vi "Add File to Tree.vi"(4 "Hide Undefined Channels":bool, 5 "Relative File Path":string, 6 "Filter Settings":T1={"Filtered Groups"=[], "Group Filter Mode"=enum."Exclude", "Group Filter Regex?"=FALSE, "Filtered Channels"=[], "Channel Filter Mode"=enum."Exclude", "Channel Filter Regex?"=FALSE, "Filter Time Start"=timestamp(0 s since 1904-01-01), "Filter Time End"=timestamp(0 s since 1904-01-01), "Time Filter Mode"=enum."Include", "Time Filter Enabled"=FALSE}, 7 "Hierarchy":string[](array[string]), 8 "error in (no error)":errorcluster, 9 "Tree Items Created In":variant, 10 "File Path":path, 11 "TreeControl in":refnum<vi>) -> (0 "error out":errorcluster, 1 "Tree Items Created Out":variant)   [LabVIEW 2017, in "XTree.xctl"]
doc: "Adds a single file to the tree. A variant is used to keep track of tree locations which have been created."
uses:
  <vilib>/addons/_NIFileIO/XTree/XTree.xctl
  <vilib>/addons/_NIFileIO/XTree/Controls/Filter Settings.ctl
  <vilib>/addons/_NIFileIO/XTree/Controls/Filter Mode.ctl
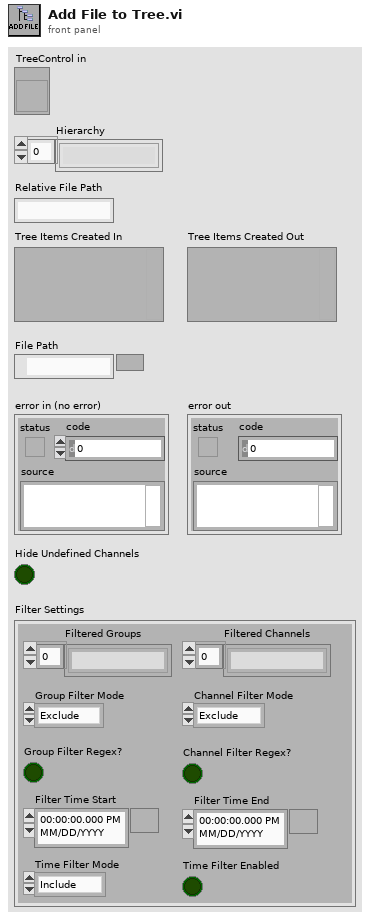
[diagram p1: front panel]
types:
  T1 = typedef "XTree.xctl/Filter Settings.ctl" = cluster{"Filtered Groups":string[], "Group Filter Mode":T2, "Group Filter Regex?":bool, "Filtered Channels":string[], "Channel Filter Mode":T2, "Channel Filter Regex?":bool, "Filter Time Start":timestamp, "Filter Time End":timestamp, "Time Filter Mode":T2, "Time Filter Enabled":bool}
  T2 = typedef "XTree.xctl/Filter Mode.ctl" = enum16{"Exclude", "Include"}
  T3 = enum16{"open", "open or create", "create or replace", "create", "open (read-only)"}
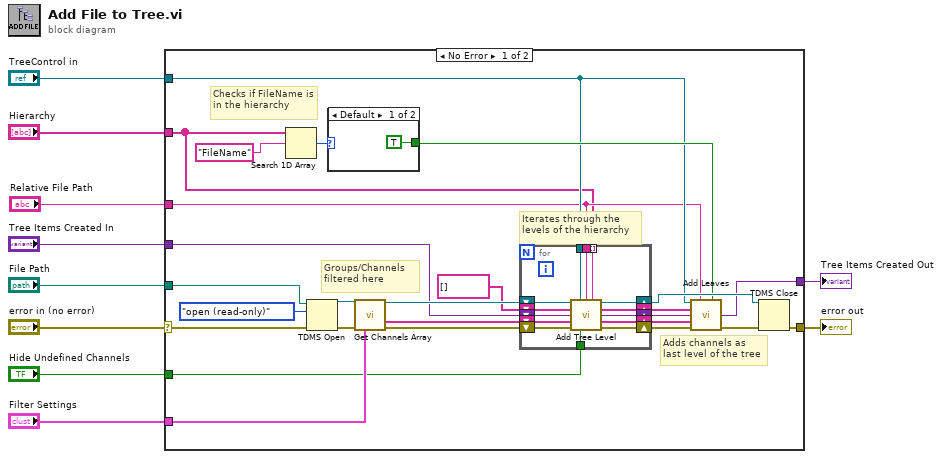
[diagram p0: block diagram]
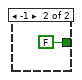
[diagram p2: hidden frame]
diagram:
  n1 = case shown="No Error" "error in (no error)" {
    selector: "error in (no error)" -> [w28 w54]
    tunnel: [w27 w54] -> w9
    tunnel: [w17 w53] -> w2
    tunnel: "Tree Items Created In" -> [w26 w53]
    tunnel: "File Path" -> [w14 _]
    tunnel: "Hierarchy" -> [w11 _]
    tunnel: "TreeControl in" -> [w19 _]
    tunnel: "Filter Settings" -> [w16 _]
    tunnel: "Hide Undefined Channels" -> [w15 _]
    tunnel: "Relative File Path" -> [w12 _]
    frame No Error {
      # "Groups/Channels filtered here"
      # "Adds channels as last level of the tree"
      # "Iterates through the levels of the hierarchy"
      # "Checks if FileName is in the hierarchy"
      n2 = Search 1D Array(1D array=w11, element="FileName") -> (index of element=w21:i32)  [unwired: 1 in]
      n3 = TDMS Open(8:w28, 10:T3."open (read-only)" ("operation (0:open)"), 11:w14) -> (0:w33:errorcluster, 3:w32:refnum<k34>)  [unwired: 4 in]
      n4 = case shown="Default" w21 {
        tunnel: [TRUE FALSE] -> w20
        frame Default {
        }
        frame -1 {
        }
      }
      n5 = call <vilib>:"Get Channels Array.vi"("TDMS File Reference in"=w32, "error in (no error)"=w33, "Filtering Settings"=w16) -> ("TDMS File Reference out"=w34:refnum<k34>, "Group/Channel Names"=w36:string[], "error out"=w13:errorcluster)  [unwired: 10 in]
      n6 = for {
        tunnel: w19 -> [w45]
        tunnel: w11 -> [w44] mode=indexing
        tunnel: w15 -> [w41]
        shift-right: [w52] -> w35
        shift-left: w34 -> [w49]
        shift-right: [w42] -> w24
        shift-left: string[] [] -> [w48]
        shift-right: [w46] -> w23
        shift-left: w26 -> [w47]
        shift-right: [w40] -> w18
        shift-left: w36 -> [w43]
        shift-right: [w50] -> w29
        shift-left: w13 -> [w51]
        tunnel: w12 -> [w39]
        n7 = call <vilib>:"Add Tree Level.vi"("tdms file"=w49, "Tree Refnum"=w45, "Relative File Path"=w39, "Property Name"=w44, "Tree Parent Tags In"=w48, "Tree Items Created In"=w47, "Group/Channel Names In"=w43, "error in (no error)"=w51, "Hide Undefined Channels"=w41) -> ("tdms file out"=w52:refnum<k34>, "Tree Parent Tags Out"=w42:string[], "Tree Items Created Out"=w46:variant, "Group/Channel Names Out"=w40:string[], "error out"=w50:errorcluster)  [unwired: 2 in]
      }
      n8 = call <vilib>:"Add Leaves.vi"("TreeControl in"=w19, "Relative File Path"=w12, "FileName In Hierarchy?"=w20, "Tree Parent Tags"=w24, "Tree Items Created In"=w23, "Group/Channel Names"=w18, "error in (no error)"=w29) -> ("Tree Items Created Out"=w17:variant, "error out"=w30:errorcluster)  [unwired: 7 in]
      n9 = TDMS Close(8:w30, 11:w35) -> (0:w27:errorcluster)  [unwired: 1 out]
    }
    frame Error {
    }
  }
  "error out" <- w9
  "Tree Items Created Out" <- w2
